vi "3 Mirrors Convert ROI.vi"(7 "Global Rectangle":i32[](array[numeric])) -> (4 "X Width (px)":dbl, 6 "X Center (px)":dbl, 8 "Y Width (px)":dbl, 10 "Y Center (px)":dbl)   [LabVIEW 2020]
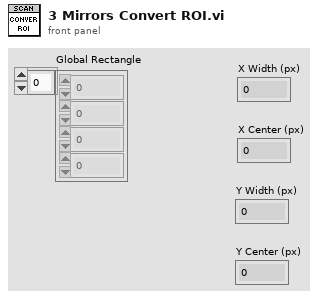
[diagram p1: front panel]
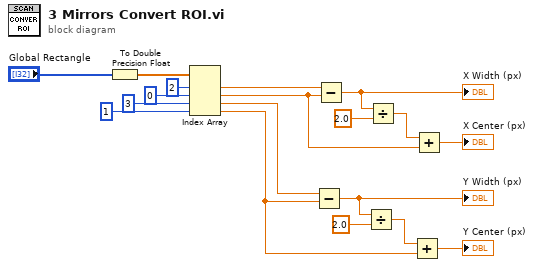
[diagram p0: block diagram]
diagram:
  n1 = To Double Precision Float(number="Global Rectangle") -> (double precision float=w14:dbl[])
  n2 = Index Array(array=w14, index #1=2 ("index"), index #2=0 ("index"), index #3=3 ("index"), index #4=1 ("index")) -> (element #1=w15:dbl, element #2=w11:dbl, element #3=w2:dbl, element #4=w1:dbl)
  n3 = Subtract(x=w2, y=w1) -> (x-y=w6:dbl)
  "Y Width (px)" <- w6
  n4 = Subtract(x=w15, y=w11) -> (x-y=w9:dbl)
  "X Width (px)" <- w9
  n5 = Divide(x=w6, y=2.0) -> (x/y=w4:dbl)
  n6 = Divide(x=w9, y=2.0) -> (x/y=w12:dbl)
  n7 = Add(x=w4, y=w1) -> (x+y=→"Y Center (px)":dbl)
  n8 = Add(x=w12, y=w11) -> (x+y=→"X Center (px)":dbl)
